vi "shuffle.vi"(1 "Array IN":variant[](array[variant])) -> (0 "Array OUT":variant[](array[variant]))   [LabVIEW 2017, in "tools.lvlib"]
uses:
  tools.lvlib
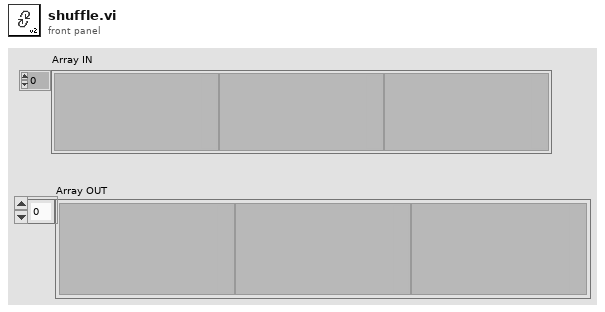
[diagram p1: front panel]
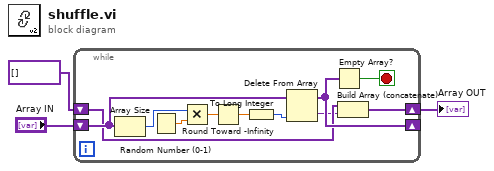
[diagram p0: block diagram]
diagram:
  n1 = while {
    shift-right: [w14] -> _
    shift-left: "Array IN" -> [w12]
    shift-right: [w8] -> w2
    shift-left: variant[] [] -> [w10]
    stop <- w13 stop-if-true
    n2 = Array Size(array=w12) -> (size(s)=w4:i32)
    n3 = Random Number (0-1)() -> (number: 0 to 1=w11:dbl)
    n4 = Multiply(x=w4, y=w11) -> (x*y=w7:dbl)
    n5 = Round Toward -Infinity(1:w7) -> (0:w6:dbl)
    n6 = To Long Integer(number=w6) -> (32bit integer=w5:i32)
    n7 = Delete From Array(array=w12, index=w5) -> (deleted portion=w9:variant, array with subset deleted=w14:variant[])  [unwired: 1 in]
    n8 = Empty Array?(array=w14) -> (empty?=w13:bool)
    n9 = Build Array (concatenate)(w10, w9) -> (w8:variant[])
  }
  "Array OUT" <- w2
